vi "CTRE_Phoenix_CANcoder_GetFaults.vi"(8 "error in":errorcluster, 11 "CTRE_CANcoder_DeviceRef":T1) -> (0 "error out":errorcluster, 2 "Faults":T2, 3 "CTRE_CANcoder_DeviceRef":T1)   [LabVIEW 2019]
doc: "Gets the current fault status of the CANcoder."
uses:
  <vilib>/Rock Robotics/WPI/ThirdParty/Phoenix-LabVIEW/CANCoder/Controls/CTRE_Phoenix_CANcoder_Faults.ctl
  <vilib>/Rock Robotics/WPI/ThirdParty/Phoenix-LabVIEW/CANCoder/Controls/CTRE_Phoenix_CANcoder_DeviceRef.ctl
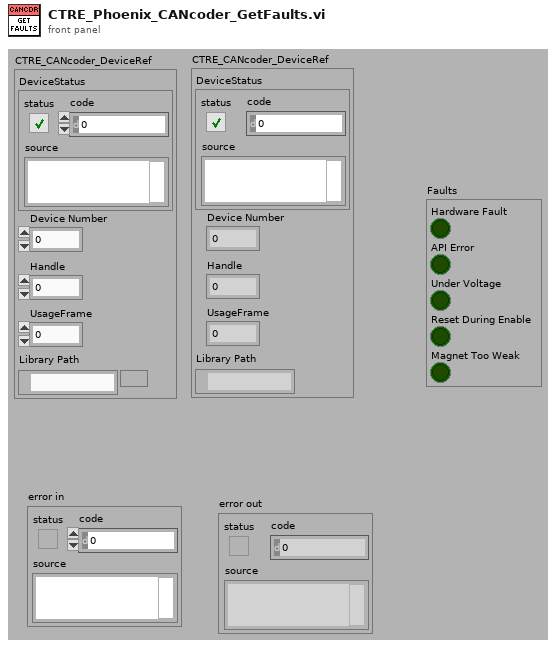
[diagram p1: front panel]
types:
  T1 = typedef "CTRE_Phoenix_CANcoder_DeviceRef.ctl" = cluster{"DeviceStatus":errorcluster, "Device Number":u8, "Handle":u64, "UsageFrame":u32, "Library Path":path}
  T2 = typedef "CTRE_Phoenix_CANcoder_Faults.ctl" = cluster{"Hardware Fault":bool, "API Error":bool, "Under Voltage":bool, "Reset During Enable":bool, "Magnet Too Weak":bool}
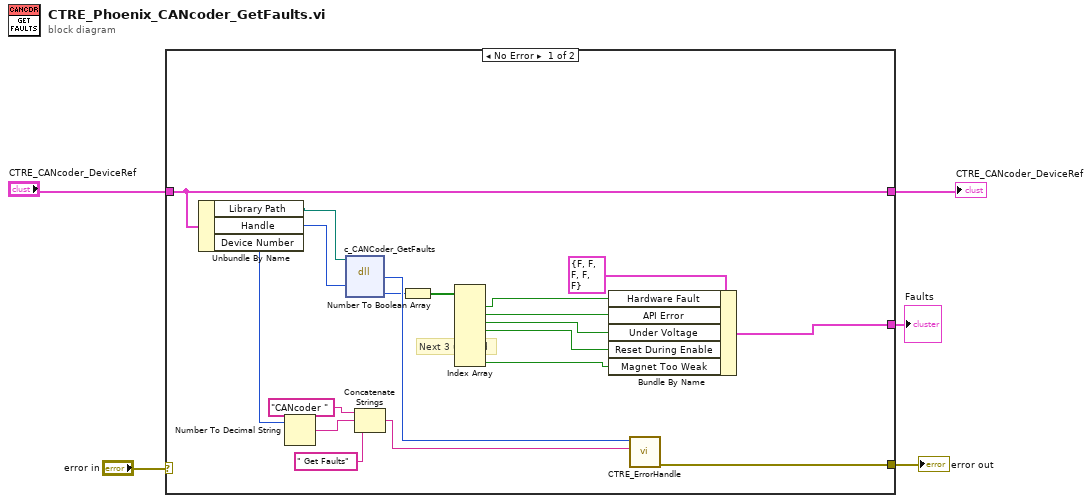
[diagram p0: block diagram]
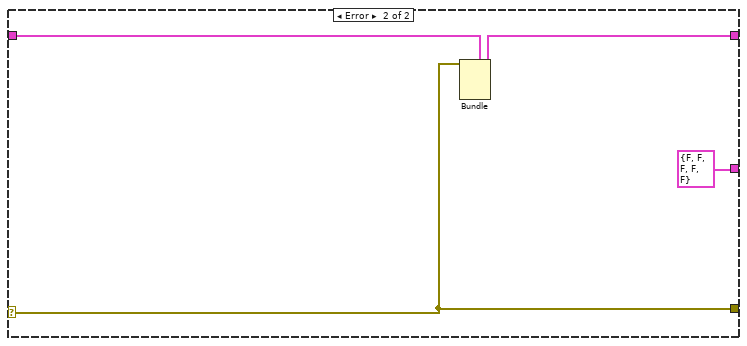
[diagram p2: hidden frame]
diagram:
  n1 = case shown="No Error" "error in" {
    selector: "error in" -> [_ w27]
    tunnel: "CTRE_CANcoder_DeviceRef" -> [w13 w28]
    tunnel: [w24 w27] -> w5
    tunnel: [w13 w26] -> w1
    tunnel: [w16 T2 {"Hardware Fault"=FALSE, "API Error"=FALSE, "Under Voltage"=FALSE, "Reset During Enable"=FALSE, "Magnet Too Weak"=FALSE} ("Faults 2")] -> w3
    frame No Error {
      # "Next 3 unused"
      n2 = Unbundle By Name(w13) -> ("Library Path"=w12:path, "Handle"=w11:u64, "Device Number"=w10:u8)
      n3 = Number To Decimal String(number=w10) -> (decimal integer string=w15:string)  [unwired: 1 in]
      n4 = dll-call lib="?" fn="c_CANCoder_GetFaults"(path in=w12, "handle"=w11) -> ("ErrorCode"=w23:i32, "faults"=w22:i32)  [unwired: 4 in, 2 out]
      n5 = Concatenate Strings("CANcoder " ("string"), w15, " Get Faults" ("string")) -> (w9:string)
      n6 = Number To Boolean Array(number=w22) -> (Boolean array=w21:bool[])
      n7 = Index Array(array=w21) -> (element #1=w20:bool, element #2=w19:bool, element #3=w18:bool, element #4=w17:bool, element #8=w7:bool)  [unwired: 8 in, 3 out]
      n8 = Bundle By Name(cluster=T2 {"Hardware Fault"=FALSE, "API Error"=FALSE, "Under Voltage"=FALSE, "Reset During Enable"=FALSE, "Magnet Too Weak"=FALSE} ("Faults 2"), "Hardware Fault"=w20, "API Error"=w19, "Under Voltage"=w18, "Reset During Enable"=w17, "Magnet Too Weak"=w7) -> (w16:T2)
      n9 = call <vilib>:"CTRE_ErrorHandle.vi"("origin"=w9, "code"=w23) -> ("error out"=w24:errorcluster)  [unwired: 9 in]
    }
    frame Error {
      n10 = Bundle(cluster=w28, "DeviceStatus"=w27) -> (w26:T1)  [unwired: 4 in]
    }
  }
  "error out" <- w5
  "Faults" <- w3
  "CTRE_CANcoder_DeviceRef" <- w1
